vi "svfa_Scaled Time Domain Window (Array).vi"(0 "input signal":dbl[](array[numeric]), 5 "window":T1 items=["None"=0, "Hanning"=1, "Hamming"=2, "Blackman-Harris"=3, "Exact Blackman"=4, "Blackman"=5, "Flat Top"=6, "4 Term B-Harris "=7, "7 Term B-Harris"=8, "Low Sidelobe"=9, "Force"=64, "Exponential"=65, "Blackman Nuttall"=11, "Triangle"=30, "Bartlett-Hanning"=31, "Bohman"=32, "Parzen"=33, "Welch"=34, "Kaiser"=60, "Dolph-Chebyshev"=61, "Gaussian"=62], 7 "window parameter":dbl=nan format="%0.2f", 11 "error in":errorcluster) -> (4 "windowed signal":dbl[](array[numeric]), 6 "dup window":T1 items=["None"=0, "Hanning"=1, "Hamming"=2, "Blackman-Harris"=3, "Exact Blackman"=4, "Blackman"=5, "Flat Top"=6, "4 Term B-Harris "=7, "7 Term B-Harris"=8, "Low Sidelobe"=9, "Force"=64, "Exponential"=65, "Blackman Nuttall"=11, "Triangle"=30, "Bartlett-Hanning"=31, "Bohman"=32, "Parzen"=33, "Welch"=34, "Kaiser"=60, "Dolph-Chebyshev"=61, "Gaussian"=62], 8 "window length":i32, 10 "FFT length":i32, 13 "window constants":cluster{"ENBW":dbl, "CG":dbl} {"CG" format="%.2f"; "ENBW" format="%.2f"}, 15 "error out":errorcluster)   [LabVIEW 2017]
doc: "Applies the selected window to the time-domain signal. The VI scales the result so that when the power or amplitude spectrum of the windowed waveform is computed, all windows provide the same level within the accuracy constraints of the window."
uses:
  <vilib>/addons/_NISVFA/_Shared subVIs/Controls/svc_Window.ctl
  <vilib>/Analysis/4window.llb/Force Window (DBL).vi
  <vilib>/Analysis/4window.llb/Exponential Window (DBL).vi
  <vilib>/Analysis/0measdsp.llb/Scaled Time Domain Window (DBL).vi
  <vilib>/Analysis/NI_AALPro.lvlib
panel:
  # "Scaled Time Domain Window"
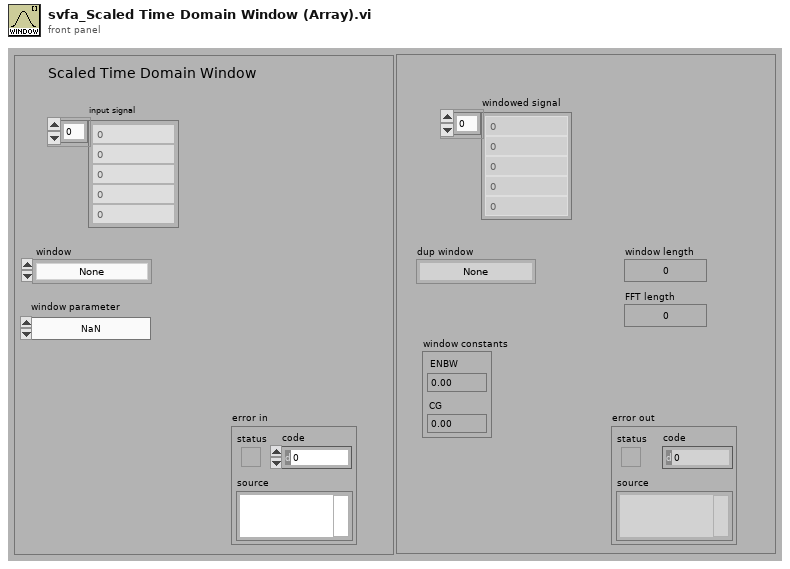
[diagram p1: front panel]
types:
  T1 = typedef "svc_Window.ctl" = u32
  T2 = typedef "NI_AALPro.lvlib/windowTd.ctl" = u32
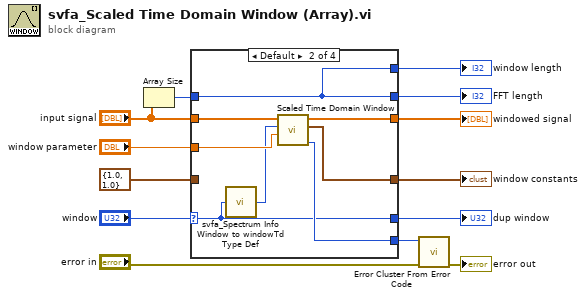
[diagram p0: block diagram]
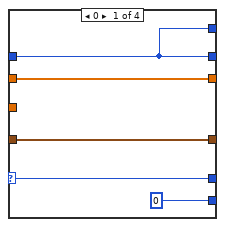
[diagram p2: hidden frame]
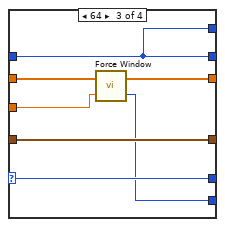
[diagram p3: hidden frame]
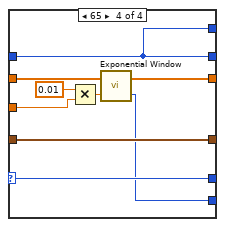
[diagram p4: hidden frame]
diagram:
  n1 = Array Size(array="input signal") -> (size(s)=w6:i32)
  n2 = case shown="Default" "window" {
    selector: "window" -> [w16 w20 w31 w38]
    tunnel: [w17 w25 w28 w35] -> w7
    tunnel: [w18 w22 w29 w36] -> w4
    tunnel: [w15 w26 w32 w39] -> w11
    tunnel: [w16 w20 w31 w38] -> w12
    tunnel: "window parameter" -> [_ w24 w33 w42]
    tunnel: cluster{"eq noise BW":dbl, "coherent gain":dbl} {"eq noise BW"=1.0, "coherent gain"=1.0} ("window properties") -> [w17 _ w28 w35]
    tunnel: [w15 w26 w32 w39] -> w9
    tunnel: "input signal" -> [w18 w23 w30 w37]
    tunnel: w6 -> [w15 w26 w32 w39]
    tunnel: [0 ("error") w21 w27 w34] -> w3
    frame 0 {
    }
    frame Default {
      n3 = call <vilib>:"svfa_Spectrum Info Window to windowTd Type Def.vi"("window"=w20) -> ("window"=w19:T2)  [unwired: 4 in]
      n4 = call-poly <vilib>:"Scaled Time Domain Window.vi"("window parameter"=w24, "window"=w19, "X"=w23) -> ("error"=w21:i32, "window properties"=w25:cluster{"eq noise BW":dbl, "coherent gain":dbl}, "Windowed X"=w22:dbl[])  [unwired: 6 in]
    }
    frame 64 {
      n5 = call-poly <vilib>:"Force Window.vi"("duty cycle(%)"=w33, "X"=w30) -> ("error"=w27:i32, "Windowed X"=w29:dbl[])
    }
    frame 65 {
      n6 = Multiply(x=0.01 ("y"), y=w42) -> (x*y=w40:dbl)
      n7 = call-poly <vilib>:"Exponential Window.vi"("final value"=w40, "X"=w37) -> ("error"=w34:i32, "Windowed X"=w36:dbl[])
    }
  }
  "window constants" <- w7
  "windowed signal" <- w4
  "window length" <- w11
  "dup window" <- w12
  "FFT length" <- w9
  n8 = call <vilib>:"Error Cluster From Error Code.vi"("error in (no error)"="error in", "error code (0)"=w3) -> ("error out"=→"error out":errorcluster)  [unwired: 7 in]
